vi "listMessageFiles.vi"(11 "folder Path":path) -> (1 "All Files in Dir":path[](array[path])=[path "/Volumes/CentralDataCache/2021/GDW-Metadata/metadata/Logs/Logs_01-2021/01-01/D01-Messages.xls", path "/Volumes/CentralDataCache/2021/GDW-Metadata/metadata/Logs/Logs_01-2021/02-01/D02-Messages.xls", path "/Volumes/CentralDataCache/2021/GDW-Metadata/metadata/Logs/Logs_01-2021/03-01/D03-Messages.xls", path "/Volumes/CentralDataCache/2021/GDW-Metadata/metadata/Logs/Logs_01-2021/04-01/D04-Messages.xls", path "/Volumes/CentralDataCache/2021/GDW-Metadata/metadata/Logs/Logs_01-2021/05-01/D05-Messages.xls", path "/Volumes/CentralDataCache/2021/GDW-Metadata/metadata/Logs/Logs_01-2021/06-01/D06-Messages.xls", path "/Volumes/CentralDataCache/2021/GDW-Metadata/metadata/Logs/Logs_01-2021/07-01/D07-Messages.xls", path "/Volumes/CentralDataCache/2021/GDW-Metadata/metadata/Logs/Logs_01-2021/08-01/D08-Messages.xls", path "/Volumes/CentralDataCache/2021/GDW-Metadata/metadata/Logs/Logs_01-2021/09-01/D09-Messages.xls", path "/Volumes/CentralDataCache/2021/GDW-Metadata/metadata/Logs/Logs_01-2021/10-01/D10-Messages.xls", path "/Volumes/CentralDataCache/2021/GDW-Metadata/metadata/Logs/Logs_01-2021/11-01/D11-Messages.xls", path "/Volumes/CentralDataCache/2021/GDW-Metadata/metadata/Logs/Logs_01-2021/12-01/D12-Messages.xls", path "/Volumes/CentralDataCache/2021/GDW-Metadata/metadata/Logs/Logs_01-2021/13-01/D13-Messages.xls", path "/Volumes/CentralDataCache/2021/GDW-Metadata/metadata/Logs/Logs_01-2021/14-01/D14-Messages.xls", path "/Volumes/CentralDataCache/2021/GDW-Metadata/metadata/Logs/Logs_01-2021/15-01/D15-Messages.xls", path "/Volumes/CentralDataCache/2021/GDW-Metadata/metadata/Logs/Logs_01-2021/16-01/D16-Messages.xls", path "/Volumes/CentralDataCache/2021/GDW-Metadata/metadata/Logs/Logs_01-2021/17-01/D17-Messages.xls", path "/Volumes/CentralDataCache/2021/GDW-Metadata/metadata/Logs/Logs_01-2021/18-01/D18-Messages.xls", path "/Volumes/CentralDataCache/2021/GDW-Metadata/metadata/Logs/Logs_01-2021/19-01/D19-Messages.xls", path "/Volumes/CentralDataCache/2021/GDW-Metadata/metadata/Logs/Logs_01-2021/20-01/D20-Messages.xls", path "/Volumes/CentralDataCache/2021/GDW-Metadata/metadata/Logs/Logs_01-2021/21-01/D21-Messages.xls", path "/Volumes/CentralDataCache/2021/GDW-Metadata/metadata/Logs/Logs_01-2021/22-01/D22-Messages.xls", path "/Volumes/CentralDataCache/2021/GDW-Metadata/metadata/Logs/Logs_01-2021/23-01/D23-Messages.xls", path "/Volumes/CentralDataCache/2021/GDW-Metadata/metadata/Logs/Logs_01-2021/24-01/D24-Messages.xls", path "/Volumes/CentralDataCache/2021/GDW-Metadata/metadata/Logs/Logs_01-2021/25-01/D25-Messages.xls", path "/Volumes/CentralDataCache/2021/GDW-Metadata/metadata/Logs/Logs_01-2021/26-01/D26-Messages.xls", path "/Volumes/CentralDataCache/2021/GDW-Metadata/metadata/Logs/Logs_01-2021/27-01/D27-Messages.xls", path "/Volumes/CentralDataCache/2021/GDW-Metadata/metadata/Logs/Logs_01-2021/28-01/D28-Messages.xls", path "/Volumes/CentralDataCache/2021/GDW-Metadata/metadata/Logs/Logs_01-2021/29-01/D29-Messages.xls", path "/Volumes/CentralDataCache/2021/GDW-Metadata/metadata/Logs/Logs_01-2021/30-01/D30-Messages.xls", path "/Volumes/CentralDataCache/2021/GDW-Metadata/metadata/Logs/Logs_01-2021/31-01/D31-Messages.xls", path "/Volumes/CentralDataCache/2021/GDW-Metadata/metadata/Logs/Logs_02-2021/01-02/D01-Messages.xls", path "/Volumes/CentralDataCache/2021/GDW-Metadata/metadata/Logs/Logs_02-2021/02-02/D02-Messages.xls", path "/Volumes/CentralDataCache/2021/GDW-Metadata/metadata/Logs/Logs_02-2021/03-02/D03-Messages.xls", path "/Volumes/CentralDataCache/2021/GDW-Metadata/metadata/Logs/Logs_02-2021/04-02/D04-Messages.xls", path "/Volumes/CentralDataCache/2021/GDW-Metadata/metadata/Logs/Logs_02-2021/05-02/D05-Messages.xls", path "/Volumes/CentralDataCache/2021/GDW-Metadata/metadata/Logs/Logs_02-2021/06-02/D06-Messages.xls", path "/Volumes/CentralDataCache/2021/GDW-Metadata/metadata/Logs/Logs_02-2021/07-02/D07-Messages.xls", path "/Volumes/CentralDataCache/2021/GDW-Metadata/metadata/Logs/Logs_02-2021/08-02/D08-Messages.xls", path "/Volumes/CentralDataCache/2021/GDW-Metadata/metadata/Logs/Logs_02-2021/09-02/D09-Messages.xls", path "/Volumes/CentralDataCache/2021/GDW-Metadata/metadata/Logs/Logs_02-2021/10-02/D10-Messages.xls", path "/Volumes/CentralDataCache/2021/GDW-Metadata/metadata/Logs/Logs_02-2021/11-02/D11-Messages.xls", path "/Volumes/CentralDataCache/2021/GDW-Metadata/metadata/Logs/Logs_02-2021/12-02/D12-Messages.xls", path "/Volumes/CentralDataCache/2021/GDW-Metadata/metadata/Logs/Logs_02-2021/13-02/D13-Messages.xls", path "/Volumes/CentralDataCache/2021/GDW-Metadata/metadata/Logs/Logs_02-2021/14-02/D14-Messages.xls", path "/Volumes/CentralDataCache/2021/GDW-Metadata/metadata/Logs/Logs_02-2021/15-02/D15-Messages.xls", path "/Volumes/CentralDataCache/2021/GDW-Metadata/metadata/Logs/Logs_02-2021/16-02/D16-Messages.xls", path "/Volumes/CentralDataCache/2021/GDW-Metadata/metadata/Logs/Logs_02-2021/17-02/D17-Messages.xls", path "/Volumes/CentralDataCache/2021/GDW-Metadata/metadata/Logs/Logs_02-2021/18-02/D18-Messages.xls", path "/Volumes/CentralDataCache/2021/GDW-Metadata/metadata/Logs/Logs_02-2021/19-02/D19-Messages.xls", path "/Volumes/CentralDataCache/2021/GDW-Metadata/metadata/Logs/Logs_02-2021/20-02/D20-Messages.xls", path "/Volumes/CentralDataCache/2021/GDW-Metadata/metadata/Logs/Logs_02-2021/21-02/D21-Messages.xls", path "/Volumes/CentralDataCache/2021/GDW-Metadata/metadata/Logs/Logs_02-2021/22-02/D22-Messages.xls", path "/Volumes/CentralDataCache/2021/GDW-Metadata/metadata/Logs/Logs_02-2021/23-02/D23-Messages.xls", path "/Volumes/CentralDataCache/2021/GDW-Metadata/metadata/Logs/Logs_02-2021/24-02/D24-Messages.xls", path "/Volumes/CentralDataCache/2021/GDW-Metadata/metadata/Logs/Logs_02-2021/25-02/D25-Messages.xls", path "/Volumes/CentralDataCache/2021/GDW-Metadata/metadata/Logs/Logs_02-2021/26-02/D26-Messages.xls", path "/Volumes/CentralDataCache/2021/GDW-Metadata/metadata/Logs/Logs_02-2021/27-02/D27-Messages.xls", path "/Volumes/CentralDataCache/2021/GDW-Metadata/metadata/Logs/Logs_02-2021/28-02/D28-Messages.xls", path "/Volumes/CentralDataCache/2021/GDW-Metadata/metadata/Logs/Logs_03-2021/01-03/D01-Messages.xls", path "/Volumes/CentralDataCache/2021/GDW-Metadata/metadata/Logs/Logs_03-2021/02-03/D02-Messages.xls", path "/Volumes/CentralDataCache/2021/GDW-Metadata/metadata/Logs/Logs_03-2021/03-03/D03-Messages.xls", path "/Volumes/CentralDataCache/2021/GDW-Metadata/metadata/Logs/Logs_03-2021/04-03/D04-Messages.xls", path "/Volumes/CentralDataCache/2021/GDW-Metadata/metadata/Logs/Logs_03-2021/05-03/D05-Messages.xls", path "/Volumes/CentralDataCache/2021/GDW-Metadata/metadata/Logs/Logs_03-2021/06-03/D06-Messages.xls", path "/Volumes/CentralDataCache/2021/GDW-Metadata/metadata/Logs/Logs_03-2021/07-03/D07-Messages.xls", path "/Volumes/CentralDataCache/2021/GDW-Metadata/metadata/Logs/Logs_03-2021/08-03/D08-Messages.xls", path "/Volumes/CentralDataCache/2021/GDW-Metadata/metadata/Logs/Logs_03-2021/09-03/D09-Messages.xls", path "/Volumes/CentralDataCache/2021/GDW-Metadata/metadata/Logs/Logs_03-2021/10-03/D10-Messages.xls", path "/Volumes/CentralDataCache/2021/GDW-Metadata/metadata/Logs/Logs_03-2021/11-03/D11-Messages.xls", path "/Volumes/CentralDataCache/2021/GDW-Metadata/metadata/Logs/Logs_03-2021/12-03/D12-Messages.xls", path "/Volumes/CentralDataCache/2021/GDW-Metadata/metadata/Logs/Logs_03-2021/13-03/D13-Messages.xls", path "/Volumes/CentralDataCache/2021/GDW-Metadata/metadata/Logs/Logs_03-2021/14-03/D14-Messages.xls", path "/Volumes/CentralDataCache/2021/GDW-Metadata/metadata/Logs/Logs_03-2021/15-03/D15-Messages.xls", path "/Volumes/CentralDataCache/2021/GDW-Metadata/metadata/Logs/Logs_03-2021/16-03/D16-Messages.xls", path "/Volumes/CentralDataCache/2021/GDW-Metadata/metadata/Logs/Logs_03-2021/17-03/D17-Messages.xls", path "/Volumes/CentralDataCache/2021/GDW-Metadata/metadata/Logs/Logs_03-2021/18-03/D18-Messages.xls", path "/Volumes/CentralDataCache/2021/GDW-Metadata/metadata/Logs/Logs_03-2021/19-03/D19-Messages.xls", path "/Volumes/CentralDataCache/2021/GDW-Metadata/metadata/Logs/Logs_03-2021/20-03/D20-Messages.xls", path "/Volumes/CentralDataCache/2021/GDW-Metadata/metadata/Logs/Logs_03-2021/21-03/D21-Messages.xls", path "/Volumes/CentralDataCache/2021/GDW-Metadata/metadata/Logs/Logs_03-2021/22-03/D22-Messages.xls", path "/Volumes/CentralDataCache/2021/GDW-Metadata/metadata/Logs/Logs_03-2021/23-03/D23-Messages.xls", path "/Volumes/CentralDataCache/2021/GDW-Metadata/metadata/Logs/Logs_03-2021/24-03/D24-Messages.xls", path "/Volumes/CentralDataCache/2021/GDW-Metadata/metadata/Logs/Logs_03-2021/25-03/D25-Messages.xls", path "/Volumes/CentralDataCache/2021/GDW-Metadata/metadata/Logs/Logs_03-2021/26-03/D26-Messages.xls", path "/Volumes/CentralDataCache/2021/GDW-Metadata/metadata/Logs/Logs_03-2021/27-03/D27-Messages.xls", path "/Volumes/CentralDataCache/2021/GDW-Metadata/metadata/Logs/Logs_03-2021/29-03/D29-Messages.xls", path "/Volumes/CentralDataCache/2021/GDW-Metadata/metadata/Logs/Logs_03-2021/30-03/D30-Messages.xls", path "/Volumes/CentralDataCache/2021/GDW-Metadata/metadata/Logs/Logs_03-2021/31-03/D31-Messages.xls", path "/Volumes/CentralDataCache/2021/GDW-Metadata/metadata/Logs/Logs_04-2021/01-04/D01-Messages.xls", path "/Volumes/CentralDataCache/2021/GDW-Metadata/metadata/Logs/Logs_04-2021/02-04/D02-Messages.xls", path "/Volumes/CentralDataCache/2021/GDW-Metadata/metadata/Logs/Logs_04-2021/03-04/D03-Messages.xls", path "/Volumes/CentralDataCache/2021/GDW-Metadata/metadata/Logs/Logs_04-2021/04-04/D04-Messages.xls", path "/Volumes/CentralDataCache/2021/GDW-Metadata/metadata/Logs/Logs_04-2021/05-04/D05-Messages.xls", path "/Volumes/CentralDataCache/2021/GDW-Metadata/metadata/Logs/Logs_04-2021/06-04/D06-Messages.xls", path "/Volumes/CentralDataCache/2021/GDW-Metadata/metadata/Logs/Logs_04-2021/07-04/D07-Messages.xls", path "/Volumes/CentralDataCache/2021/GDW-Metadata/metadata/Logs/Logs_04-2021/08-04/D08-Messages.xls", path "/Volumes/CentralDataCache/2021/GDW-Metadata/metadata/Logs/Logs_04-2021/09-04/D09-Messages.xls", path "/Volumes/CentralDataCache/2021/GDW-Metadata/metadata/Logs/Logs_04-2021/10-04/D10-Messages.xls", path "/Volumes/CentralDataCache/2021/GDW-Metadata/metadata/Logs/Logs_04-2021/11-04/D11-Messages.xls", path "/Volumes/CentralDataCache/2021/GDW-Metadata/metadata/Logs/Logs_04-2021/12-04/D12-Messages.xls", path "/Volumes/CentralDataCache/2021/GDW-Metadata/metadata/Logs/Logs_04-2021/13-04/D13-Messages.xls", path "/Volumes/CentralDataCache/2021/GDW-Metadata/metadata/Logs/Logs_04-2021/14-04/D14-Messages.xls", path "/Volumes/CentralDataCache/2021/GDW-Metadata/metadata/Logs/Logs_04-2021/15-04/D15-Messages.xls", path "/Volumes/CentralDataCache/2021/GDW-Metadata/metadata/Logs/Logs_04-2021/16-04/D16-Messages.xls", path "/Volumes/CentralDataCache/2021/GDW-Metadata/metadata/Logs/Logs_04-2021/17-04/D17-Messages.xls", path "/Volumes/CentralDataCache/2021/GDW-Metadata/metadata/Logs/Logs_04-2021/18-04/D18-Messages.xls", path "/Volumes/CentralDataCache/2021/GDW-Metadata/metadata/Logs/Logs_04-2021/19-04/D19-Messages.xls", path "/Volumes/CentralDataCache/2021/GDW-Metadata/metadata/Logs/Logs_04-2021/20-04/D20-Messages.xls", path "/Volumes/CentralDataCache/2021/GDW-Metadata/metadata/Logs/Logs_04-2021/21-04/D21-Messages.xls", path "/Volumes/CentralDataCache/2021/GDW-Metadata/metadata/Logs/Logs_04-2021/22-04/D22-Messages.xls", path "/Volumes/CentralDataCache/2021/GDW-Metadata/metadata/Logs/Logs_04-2021/23-04/D23-Messages.xls", path "/Volumes/CentralDataCache/2021/GDW-Metadata/metadata/Logs/Logs_04-2021/24-04/D24-Messages.xls", path "/Volumes/CentralDataCache/2021/GDW-Metadata/metadata/Logs/Logs_04-2021/25-04/D25-Messages.xls", path "/Volumes/CentralDataCache/2021/GDW-Metadata/metadata/Logs/Logs_04-2021/26-04/D26-Messages.xls", path "/Volumes/CentralDataCache/2021/GDW-Metadata/metadata/Logs/Logs_04-2021/27-04/D27-Messages.xls", path "/Volumes/CentralDataCache/2021/GDW-Metadata/metadata/Logs/Logs_04-2021/28-04/D28-Messages.xls", path "/Volumes/CentralDataCache/2021/GDW-Metadata/metadata/Logs/Logs_04-2021/29-04/D29-Messages.xls", path "/Volumes/CentralDataCache/2021/GDW-Metadata/metadata/Logs/Logs_04-2021/30-04/D30-Messages.xls", path "/Volumes/CentralDataCache/2021/GDW-Metadata/metadata/Logs/Logs_05-2021/01-05/D01-Messages.xls", path "/Volumes/CentralDataCache/2021/GDW-Metadata/metadata/Logs/Logs_05-2021/02-05/D02-Messages.xls", path "/Volumes/CentralDataCache/2021/GDW-Metadata/metadata/Logs/Logs_05-2021/03-05/D03-Messages.xls", path "/Volumes/CentralDataCache/2021/GDW-Metadata/metadata/Logs/Logs_05-2021/04-05/D04-Messages.xls", path "/Volumes/CentralDataCache/2021/GDW-Metadata/metadata/Logs/Logs_05-2021/05-05/D05-Messages.xls", path "/Volumes/CentralDataCache/2021/GDW-Metadata/metadata/Logs/Logs_05-2021/06-05/D06-Messages.xls", path "/Volumes/CentralDataCache/2021/GDW-Metadata/metadata/Logs/Logs_05-2021/07-05/D07-Messages.xls", path "/Volumes/CentralDataCache/2021/GDW-Metadata/metadata/Logs/Logs_05-2021/08-05/D08-Messages.xls", path "/Volumes/CentralDataCache/2021/GDW-Metadata/metadata/Logs/Logs_05-2021/09-05/D09-Messages.xls", path "/Volumes/CentralDataCache/2021/GDW-Metadata/metadata/Logs/Logs_05-2021/10-05/D10-Messages.xls", path "/Volumes/CentralDataCache/2021/GDW-Metadata/metadata/Logs/Logs_05-2021/11-05/D11-Messages.xls", path "/Volumes/CentralDataCache/2021/GDW-Metadata/metadata/Logs/Logs_05-2021/12-05/D12-Messages.xls", path "/Volumes/CentralDataCache/2021/GDW-Metadata/metadata/Logs/Logs_05-2021/13-05/D13-Messages.xls", path "/Volumes/CentralDataCache/2021/GDW-Metadata/metadata/Logs/Logs_05-2021/14-05/D14-Messages.xls", path "/Volumes/CentralDataCache/2021/GDW-Metadata/metadata/Logs/Logs_05-2021/15-05/D15-Messages.xls", path "/Volumes/CentralDataCache/2021/GDW-Metadata/metadata/Logs/Logs_05-2021/16-05/D16-Messages.xls", path "/Volumes/CentralDataCache/2021/GDW-Metadata/metadata/Logs/Logs_05-2021/17-05/D17-Messages.xls", path "/Volumes/CentralDataCache/2021/GDW-Metadata/metadata/Logs/Logs_05-2021/18-05/D18-Messages.xls", path "/Volumes/CentralDataCache/2021/GDW-Metadata/metadata/Logs/Logs_05-2021/19-05/D19-Messages.xls", path "/Volumes/CentralDataCache/2021/GDW-Metadata/metadata/Logs/Logs_05-2021/20-05/D20-Messages.xls", path "/Volumes/CentralDataCache/2021/GDW-Metadata/metadata/Logs/Logs_05-2021/21-05/D21-Messages.xls", path "/Volumes/CentralDataCache/2021/GDW-Metadata/metadata/Logs/Logs_05-2021/22-05/D22-Messages.xls", path "/Volumes/CentralDataCache/2021/GDW-Metadata/metadata/Logs/Logs_05-2021/23-05/D23-Messages.xls", path "/Volumes/CentralDataCache/2021/GDW-Metadata/metadata/Logs/Logs_05-2021/24-05/D24-Messages.xls", path "/Volumes/CentralDataCache/2021/GDW-Metadata/metadata/Logs/Logs_05-2021/25-05/D25-Messages.xls", path "/Volumes/CentralDataCache/2021/GDW-Metadata/metadata/Logs/Logs_05-2021/26-05/D26-Messages.xls", path "/Volumes/CentralDataCache/2021/GDW-Metadata/metadata/Logs/Logs_05-2021/27-05/D27-Messages.xls", path "/Volumes/CentralDataCache/2021/GDW-Metadata/metadata/Logs/Logs_05-2021/28-05/D28-Messages.xls", path "/Volumes/CentralDataCache/2021/GDW-Metadata/metadata/Logs/Logs_05-2021/29-05/D29-Messages.xls", path "/Volumes/CentralDataCache/2021/GDW-Metadata/metadata/Logs/Logs_05-2021/30-05/D30-Messages.xls", path "/Volumes/CentralDataCache/2021/GDW-Metadata/metadata/Logs/Logs_05-2021/31-05/D31-Messages.xls", path "/Volumes/CentralDataCache/2021/GDW-Metadata/metadata/Logs/Logs_06-2021/01-06/D01-Messages.xls", path "/Volumes/CentralDataCache/2021/GDW-Metadata/metadata/Logs/Logs_06-2021/02-06/D02-Messages.xls", path "/Volumes/CentralDataCache/2021/GDW-Metadata/metadata/Logs/Logs_06-2021/03-06/D03-Messages.xls", path "/Volumes/CentralDataCache/2021/GDW-Metadata/metadata/Logs/Logs_06-2021/04-06/D04-Messages.xls", path "/Volumes/CentralDataCache/2021/GDW-Metadata/metadata/Logs/Logs_06-2021/05-06/D05-Messages.xls", path "/Volumes/CentralDataCache/2021/GDW-Metadata/metadata/Logs/Logs_06-2021/06-06/D06-Messages.xls", path "/Volumes/CentralDataCache/2021/GDW-Metadata/metadata/Logs/Logs_06-2021/07-06/D07-Messages.xls", path "/Volumes/CentralDataCache/2021/GDW-Metadata/metadata/Logs/Logs_06-2021/08-06/D08-Messages.xls", path "/Volumes/CentralDataCache/2021/GDW-Metadata/metadata/Logs/Logs_06-2021/09-06/D09-Messages.xls", path "/Volumes/CentralDataCache/2021/GDW-Metadata/metadata/Logs/Logs_06-2021/10-06/D10-Messages.xls", path "/Volumes/CentralDataCache/2021/GDW-Metadata/metadata/Logs/Logs_06-2021/11-06/D11-Messages.xls", path "/Volumes/CentralDataCache/2021/GDW-Metadata/metadata/Logs/Logs_06-2021/12-06/D12-Messages.xls", path "/Volumes/CentralDataCache/2021/GDW-Metadata/metadata/Logs/Logs_06-2021/13-06/D13-Messages.xls", path "/Volumes/CentralDataCache/2021/GDW-Metadata/metadata/Logs/Logs_06-2021/14-06/D14-Messages.xls", path "/Volumes/CentralDataCache/2021/GDW-Metadata/metadata/Logs/Logs_06-2021/15-06/D15-Messages.xls", path "/Volumes/CentralDataCache/2021/GDW-Metadata/metadata/Logs/Logs_06-2021/16-06/D16-Messages.xls", path "/Volumes/CentralDataCache/2021/GDW-Metadata/metadata/Logs/Logs_06-2021/17-06/D17-Messages.xls", path "/Volumes/CentralDataCache/2021/GDW-Metadata/metadata/Logs/Logs_06-2021/18-06/D18-Messages.xls", path "/Volumes/CentralDataCache/2021/GDW-Metadata/metadata/Logs/Logs_06-2021/19-06/D19-Messages.xls", path "/Volumes/CentralDataCache/2021/GDW-Metadata/metadata/Logs/Logs_06-2021/20-06/D20-Messages.xls", path "/Volumes/CentralDataCache/2021/GDW-Metadata/metadata/Logs/Logs_06-2021/21-06/D21-Messages.xls", path "/Volumes/CentralDataCache/2021/GDW-Metadata/metadata/Logs/Logs_06-2021/22-06/D22-Messages.xls", path "/Volumes/CentralDataCache/2021/GDW-Metadata/metadata/Logs/Logs_06-2021/23-06/D23-Messages.xls", path "/Volumes/CentralDataCache/2021/GDW-Metadata/metadata/Logs/Logs_06-2021/24-06/D24-Messages.xls", path "/Volumes/CentralDataCache/2021/GDW-Metadata/metadata/Logs/Logs_06-2021/25-06/D25-Messages.xls", path "/Volumes/CentralDataCache/2021/GDW-Metadata/metadata/Logs/Logs_06-2021/26-06/D26-Messages.xls", path "/Volumes/CentralDataCache/2021/GDW-Metadata/metadata/Logs/Logs_06-2021/27-06/D27-Messages.xls", path "/Volumes/CentralDataCache/2021/GDW-Metadata/metadata/Logs/Logs_06-2021/28-06/D28-Messages.xls", path "/Volumes/CentralDataCache/2021/GDW-Metadata/metadata/Logs/Logs_06-2021/29-06/D29-Messages.xls", path "/Volumes/CentralDataCache/2021/GDW-Metadata/metadata/Logs/Logs_06-2021/30-06/D30-Messages.xls", path "/Volumes/CentralDataCache/2021/GDW-Metadata/metadata/Logs/Logs_07-2021/01-07/D01-Messages.xls", path "/Volumes/CentralDataCache/2021/GDW-Metadata/metadata/Logs/Logs_07-2021/02-07/D02-Messages.xls", path "/Volumes/CentralDataCache/2021/GDW-Metadata/metadata/Logs/Logs_07-2021/03-07/D03-Messages.xls", path "/Volumes/CentralDataCache/2021/GDW-Metadata/metadata/Logs/Logs_07-2021/04-07/D04-Messages.xls", path "/Volumes/CentralDataCache/2021/GDW-Metadata/metadata/Logs/Logs_07-2021/05-07/D05-Messages.xls", path "/Volumes/CentralDataCache/2021/GDW-Metadata/metadata/Logs/Logs_07-2021/06-07/D06-Messages.xls", path "/Volumes/CentralDataCache/2021/GDW-Metadata/metadata/Logs/Logs_07-2021/07-07/D07-Messages.xls", path "/Volumes/CentralDataCache/2021/GDW-Metadata/metadata/Logs/Logs_07-2021/08-07/D08-Messages.xls", path "/Volumes/CentralDataCache/2021/GDW-Metadata/metadata/Logs/Logs_07-2021/09-07/D09-Messages.xls", path "/Volumes/CentralDataCache/2021/GDW-Metadata/metadata/Logs/Logs_07-2021/10-07/D10-Messages.xls", path "/Volumes/CentralDataCache/2021/GDW-Metadata/metadata/Logs/Logs_07-2021/11-07/D11-Messages.xls", path "/Volumes/CentralDataCache/2021/GDW-Metadata/metadata/Logs/Logs_07-2021/12-07/D12-Messages.xls", path "/Volumes/CentralDataCache/2021/GDW-Metadata/metadata/Logs/Logs_07-2021/13-07/D13-Messages.xls", path "/Volumes/CentralDataCache/2021/GDW-Metadata/metadata/Logs/Logs_07-2021/14-07/D14-Messages.xls", path "/Volumes/CentralDataCache/2021/GDW-Metadata/metadata/Logs/Logs_07-2021/15-07/D15-Messages.xls", path "/Volumes/CentralDataCache/2021/GDW-Metadata/metadata/Logs/Logs_07-2021/16-07/D16-Messages.xls", path "/Volumes/CentralDataCache/2021/GDW-Metadata/metadata/Logs/Logs_07-2021/17-07/D17-Messages.xls", path "/Volumes/CentralDataCache/2021/GDW-Metadata/metadata/Logs/Logs_07-2021/18-07/D18-Messages.xls", path "/Volumes/CentralDataCache/2021/GDW-Metadata/metadata/Logs/Logs_07-2021/19-07/D19-Messages.xls", path "/Volumes/CentralDataCache/2021/GDW-Metadata/metadata/Logs/Logs_07-2021/20-07/D20-Messages.xls", path "/Volumes/CentralDataCache/2021/GDW-Metadata/metadata/Logs/Logs_07-2021/21-07/D21-Messages.xls", path "/Volumes/CentralDataCache/2021/GDW-Metadata/metadata/Logs/Logs_07-2021/22-07/D22-Messages.xls", path "/Volumes/CentralDataCache/2021/GDW-Metadata/metadata/Logs/Logs_07-2021/23-07/D23-Messages.xls", path "/Volumes/CentralDataCache/2021/GDW-Metadata/metadata/Logs/Logs_07-2021/24-07/D24-Messages.xls", path "/Volumes/CentralDataCache/2021/GDW-Metadata/metadata/Logs/Logs_07-2021/25-07/D25-Messages.xls", path "/Volumes/CentralDataCache/2021/GDW-Metadata/metadata/Logs/Logs_07-2021/26-07/D26-Messages.xls", path "/Volumes/CentralDataCache/2021/GDW-Metadata/metadata/Logs/Logs_07-2021/27-07/D27-Messages.xls", path "/Volumes/CentralDataCache/2021/GDW-Metadata/metadata/Logs/Logs_07-2021/28-07/D28-Messages.xls", path "/Volumes/CentralDataCache/2021/GDW-Metadata/metadata/Logs/Logs_07-2021/29-07/D29-Messages.xls", path "/Volumes/CentralDataCache/2021/GDW-Metadata/metadata/Logs/Logs_07-2021/30-07/D30-Messages.xls", path "/Volumes/CentralDataCache/2021/GDW-Metadata/metadata/Logs/Logs_07-2021/31-07/D31-Messages.xls", path "/Volumes/CentralDataCache/2021/GDW-Metadata/metadata/Logs/Logs_08-2021/01-08/D01-Messages.xls", path "/Volumes/CentralDataCache/2021/GDW-Metadata/metadata/Logs/Logs_08-2021/02-08/D02-Messages.xls", path "/Volumes/CentralDataCache/2021/GDW-Metadata/metadata/Logs/Logs_08-2021/03-08/D03-Messages.xls", path "/Volumes/CentralDataCache/2021/GDW-Metadata/metadata/Logs/Logs_08-2021/04-08/D04-Messages.xls", path "/Volumes/CentralDataCache/2021/GDW-Metadata/metadata/Logs/Logs_08-2021/05-08/D05-Messages.xls", path "/Volumes/CentralDataCache/2021/GDW-Metadata/metadata/Logs/Logs_08-2021/06-08/D06-Messages.xls", path "/Volumes/CentralDataCache/2021/GDW-Metadata/metadata/Logs/Logs_08-2021/07-08/D07-Messages.xls", path "/Volumes/CentralDataCache/2021/GDW-Metadata/metadata/Logs/Logs_08-2021/08-08/D08-Messages.xls", path "/Volumes/CentralDataCache/2021/GDW-Metadata/metadata/Logs/Logs_08-2021/09-08/D09-Messages.xls", path "/Volumes/CentralDataCache/2021/GDW-Metadata/metadata/Logs/Logs_08-2021/10-08/D10-Messages.xls", path "/Volumes/CentralDataCache/2021/GDW-Metadata/metadata/Logs/Logs_08-2021/11-08/D11-Messages.xls", path "/Volumes/CentralDataCache/2021/GDW-Metadata/metadata/Logs/Logs_08-2021/12-08/D12-Messages.xls", path "/Volumes/CentralDataCache/2021/GDW-Metadata/metadata/Logs/Logs_08-2021/13-08/D13-Messages.xls", path "/Volumes/CentralDataCache/2021/GDW-Metadata/metadata/Logs/Logs_08-2021/17-08/D17-Messages.xls", path "/Volumes/CentralDataCache/2021/GDW-Metadata/metadata/Logs/Logs_08-2021/18-08/D18-Messages.xls", path "/Volumes/CentralDataCache/2021/GDW-Metadata/metadata/Logs/Logs_08-2021/19-08/D19-Messages.xls", path "/Volumes/CentralDataCache/2021/GDW-Metadata/metadata/Logs/Logs_08-2021/20-08/D20-Messages.xls", path "/Volumes/CentralDataCache/2021/GDW-Metadata/metadata/Logs/Logs_08-2021/21-08/D21-Messages.xls", path "/Volumes/CentralDataCache/2021/GDW-Metadata/metadata/Logs/Logs_08-2021/22-08/D22-Messages.xls", path "/Volumes/CentralDataCache/2021/GDW-Metadata/metadata/Logs/Logs_08-2021/23-08/D23-Messages.xls", path "/Volumes/CentralDataCache/2021/GDW-Metadata/metadata/Logs/Logs_08-2021/24-08/D24-Messages.xls", path "/Volumes/CentralDataCache/2021/GDW-Metadata/metadata/Logs/Logs_08-2021/25-08/D25-Messages.xls", path "/Volumes/CentralDataCache/2021/GDW-Metadata/metadata/Logs/Logs_08-2021/26-08/D26-Messages.xls", path "/Volumes/CentralDataCache/2021/GDW-Metadata/metadata/Logs/Logs_08-2021/27-08/D27-Messages.xls", path "/Volumes/CentralDataCache/2021/GDW-Metadata/metadata/Logs/Logs_08-2021/28-08/D28-Messages.xls", path "/Volumes/CentralDataCache/2021/GDW-Metadata/metadata/Logs/Logs_08-2021/29-08/D29-Messages.xls", path "/Volumes/CentralDataCache/2021/GDW-Metadata/metadata/Logs/Logs_08-2021/30-08/D30-Messages.xls", path "/Volumes/CentralDataCache/2021/GDW-Metadata/metadata/Logs/Logs_08-2021/31-08/D31-Messages.xls", path "/Volumes/CentralDataCache/2021/GDW-Metadata/metadata/Logs/Logs_09-2021/01-09/D01-Messages.xls", path "/Volumes/CentralDataCache/2021/GDW-Metadata/metadata/Logs/Logs_09-2021/02-09/D02-Messages.xls", path "/Volumes/CentralDataCache/2021/GDW-Metadata/metadata/Logs/Logs_09-2021/03-09/D03-Messages.xls", path "/Volumes/CentralDataCache/2021/GDW-Metadata/metadata/Logs/Logs_09-2021/04-09/D04-Messages.xls", path "/Volumes/CentralDataCache/2021/GDW-Metadata/metadata/Logs/Logs_09-2021/05-09/D05-Messages.xls", path "/Volumes/CentralDataCache/2021/GDW-Metadata/metadata/Logs/Logs_09-2021/06-09/D06-Messages.xls", path "/Volumes/CentralDataCache/2021/GDW-Metadata/metadata/Logs/Logs_09-2021/07-09/D07-Messages.xls", path "/Volumes/CentralDataCache/2021/GDW-Metadata/metadata/Logs/Logs_09-2021/08-09/D08-Messages.xls", path "/Volumes/CentralDataCache/2021/GDW-Metadata/metadata/Logs/Logs_09-2021/09-09/D09-Messages.xls", path "/Volumes/CentralDataCache/2021/GDW-Metadata/metadata/Logs/Logs_09-2021/10-09/D10-Messages.xls", path "/Volumes/CentralDataCache/2021/GDW-Metadata/metadata/Logs/Logs_09-2021/11-09/D11-Messages.xls", path "/Volumes/CentralDataCache/2021/GDW-Metadata/metadata/Logs/Logs_09-2021/12-09/D12-Messages.xls", path "/Volumes/CentralDataCache/2021/GDW-Metadata/metadata/Logs/Logs_09-2021/13-09/D13-Messages.xls", path "/Volumes/CentralDataCache/2021/GDW-Metadata/metadata/Logs/Logs_09-2021/14-09/D14-Messages.xls", path "/Volumes/CentralDataCache/2021/GDW-Metadata/metadata/Logs/Logs_09-2021/15-09/D15-Messages.xls", path "/Volumes/CentralDataCache/2021/GDW-Metadata/metadata/Logs/Logs_09-2021/16-09/D16-Messages.xls", path "/Volumes/CentralDataCache/2021/GDW-Metadata/metadata/Logs/Logs_09-2021/17-09/D17-Messages.xls", path "/Volumes/CentralDataCache/2021/GDW-Metadata/metadata/Logs/Logs_09-2021/18-09/D18-Messages.xls", path "/Volumes/CentralDataCache/2021/GDW-Metadata/metadata/Logs/Logs_09-2021/19-09/D19-Messages.xls", path "/Volumes/CentralDataCache/2021/GDW-Metadata/metadata/Logs/Logs_09-2021/20-09/D20-Messages.xls", path "/Volumes/CentralDataCache/2021/GDW-Metadata/metadata/Logs/Logs_09-2021/21-09/D21-Messages.xls", path "/Volumes/CentralDataCache/2021/GDW-Metadata/metadata/Logs/Logs_09-2021/22-09/D22-Messages.xls", path "/Volumes/CentralDataCache/2021/GDW-Metadata/metadata/Logs/Logs_09-2021/23-09/D23-Messages.xls", path "/Volumes/CentralDataCache/2021/GDW-Metadata/metadata/Logs/Logs_09-2021/24-09/D24-Messages.xls", path "/Volumes/CentralDataCache/2021/GDW-Metadata/metadata/Logs/Logs_09-2021/25-09/D25-Messages.xls", path "/Volumes/CentralDataCache/2021/GDW-Metadata/metadata/Logs/Logs_09-2021/26-09/D26-Messages.xls", path "/Volumes/CentralDataCache/2021/GDW-Metadata/metadata/Logs/Logs_09-2021/27-09/D27-Messages.xls", path "/Volumes/CentralDataCache/2021/GDW-Metadata/metadata/Logs/Logs_09-2021/28-09/D28-Messages.xls", path "/Volumes/CentralDataCache/2021/GDW-Metadata/metadata/Logs/Logs_09-2021/29-09/D29-Messages.xls", path "/Volumes/CentralDataCache/2021/GDW-Metadata/metadata/Logs/Logs_09-2021/30-09/D30-Messages.xls", path "/Volumes/CentralDataCache/2021/GDW-Metadata/metadata/Logs/Logs_10-2021/01-10/D01-Messages.xls", path "/Volumes/CentralDataCache/2021/GDW-Metadata/metadata/Logs/Logs_10-2021/02-10/D02-Messages.xls", path "/Volumes/CentralDataCache/2021/GDW-Metadata/metadata/Logs/Logs_10-2021/03-10/D03-Messages.xls", path "/Volumes/CentralDataCache/2021/GDW-Metadata/metadata/Logs/Logs_10-2021/04-10/D04-Messages.xls", path "/Volumes/CentralDataCache/2021/GDW-Metadata/metadata/Logs/Logs_10-2021/05-10/D05-Messages.xls", path "/Volumes/CentralDataCache/2021/GDW-Metadata/metadata/Logs/Logs_10-2021/06-10/D06-Messages.xls", path "/Volumes/CentralDataCache/2021/GDW-Metadata/metadata/Logs/Logs_10-2021/07-10/D07-Messages.xls", path "/Volumes/CentralDataCache/2021/GDW-Metadata/metadata/Logs/Logs_10-2021/08-10/D08-Messages.xls", path "/Volumes/CentralDataCache/2021/GDW-Metadata/metadata/Logs/Logs_10-2021/09-10/D09-Messages.xls", path "/Volumes/CentralDataCache/2021/GDW-Metadata/metadata/Logs/Logs_10-2021/10-10/D10-Messages.xls", path "/Volumes/CentralDataCache/2021/GDW-Metadata/metadata/Logs/Logs_10-2021/11-10/D11-Messages.xls", path "/Volumes/CentralDataCache/2021/GDW-Metadata/metadata/Logs/Logs_10-2021/12-10/D12-Messages.xls", path "/Volumes/CentralDataCache/2021/GDW-Metadata/metadata/Logs/Logs_10-2021/13-10/D13-Messages.xls", path "/Volumes/CentralDataCache/2021/GDW-Metadata/metadata/Logs/Logs_10-2021/14-10/D14-Messages.xls", path "/Volumes/CentralDataCache/2021/GDW-Metadata/metadata/Logs/Logs_10-2021/15-10/D15-Messages.xls", path "/Volumes/CentralDataCache/2021/GDW-Metadata/metadata/Logs/Logs_10-2021/16-10/D16-Messages.xls", path "/Volumes/CentralDataCache/2021/GDW-Metadata/metadata/Logs/Logs_10-2021/17-10/D17-Messages.xls", path "/Volumes/CentralDataCache/2021/GDW-Metadata/metadata/Logs/Logs_10-2021/18-10/D18-Messages.xls", path "/Volumes/CentralDataCache/2021/GDW-Metadata/metadata/Logs/Logs_10-2021/19-10/D19-Messages.xls", path "/Volumes/CentralDataCache/2021/GDW-Metadata/metadata/Logs/Logs_10-2021/20-10/D20-Messages.xls", path "/Volumes/CentralDataCache/2021/GDW-Metadata/metadata/Logs/Logs_10-2021/21-10/D21-Messages.xls", path "/Volumes/CentralDataCache/2021/GDW-Metadata/metadata/Logs/Logs_10-2021/22-10/D22-Messages.xls", path "/Volumes/CentralDataCache/2021/GDW-Metadata/metadata/Logs/Logs_10-2021/23-10/D23-Messages.xls", path "/Volumes/CentralDataCache/2021/GDW-Metadata/metadata/Logs/Logs_10-2021/24-10/D24-Messages.xls", path "/Volumes/CentralDataCache/2021/GDW-Metadata/metadata/Logs/Logs_10-2021/25-10/D25-Messages.xls", path "/Volumes/CentralDataCache/2021/GDW-Metadata/metadata/Logs/Logs_10-2021/26-10/D26-Messages.xls"])   [LabVIEW 2020]
panel:
  in  "useCached":bool
  out "Number of Files":i32
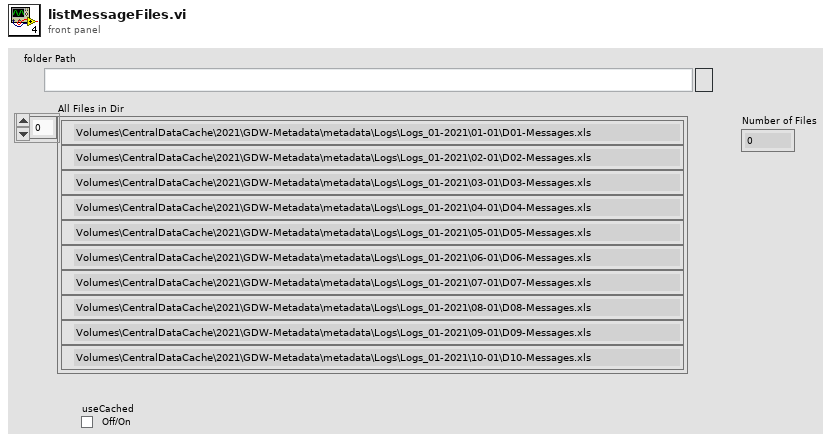
[diagram p1: front panel]
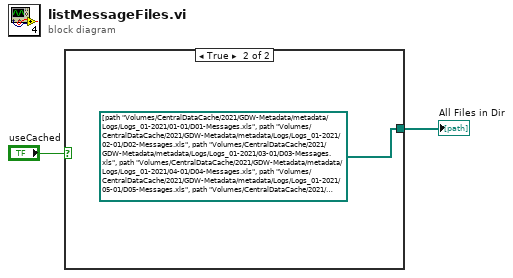
[diagram p0: block diagram]
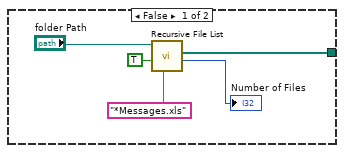
[diagram p2: hidden frame]
diagram:
  n1 = case shown="True" "useCached" {
    tunnel: [w4 path[] [path "/Volumes/CentralDataCache/2021/GDW-Metadata/metadata/Logs/Logs_01-2021/01-01/D01-Messages.xls", path "/Volumes/CentralDataCache/2021/GDW-Metadata/metadata/Logs/Logs_01-2021/02-01/D02-Messages.xls", path "/Volumes/CentralDataCache/2021/GDW-Metadata/metadata/Logs/Logs_01-2021/03-01/D03-Messages.xls", path "/Volumes/CentralDataCache/2021/GDW-Metadata/metadata/Logs/Logs_01-2021/04-01/D04-Messages.xls", path "/Volumes/CentralDataCache/2021/GDW-Metadata/metadata/Logs/Logs_01-2021/05-01/D05-Messages.xls", path "/Volumes/CentralDataCache/2021/GDW-Metadata/metadata/Logs/Logs_01-2021/06-01/D06-Messages.xls", path "/Volumes/CentralDataCache/2021/GDW-Metadata/metadata/Logs/Logs_01-2021/07-01/D07-Messages.xls", path "/Volumes/CentralDataCache/2021/GDW-Metadata/metadata/Logs/Logs_01-2021/08-01/D08-Messages.xls", path "/Volumes/CentralDataCache/2021/GDW-Metadata/metadata/Logs/Logs_01-2021/09-01/D09-Messages.xls", path "/Volumes/CentralDataCache/2021/GDW-Metadata/metadata/Logs/Logs_01-2021/10-01/D10-Messages.xls", path "/Volumes/CentralDataCache/2021/GDW-Metadata/metadata/Logs/Logs_01-2021/11-01/D11-Messages.xls", path "/Volumes/CentralDataCache/2021/GDW-Metadata/metadata/Logs/Logs_01-2021/12-01/D12-Messages.xls", path "/Volumes/CentralDataCache/2021/GDW-Metadata/metadata/Logs/Logs_01-2021/13-01/D13-Messages.xls", path "/Volumes/CentralDataCache/2021/GDW-Metadata/metadata/Logs/Logs_01-2021/14-01/D14-Messages.xls", path "/Volumes/CentralDataCache/2021/GDW-Metadata/metadata/Logs/Logs_01-2021/15-01/D15-Messages.xls", path "/Volumes/CentralDataCache/2021/GDW-Metadata/metadata/Logs/Logs_01-2021/16-01/D16-Messages.xls", path "/Volumes/CentralDataCache/2021/GDW-Metadata/metadata/Logs/Logs_01-2021/17-01/D17-Messages.xls", path "/Volumes/CentralDataCache/2021/GDW-Metadata/metadata/Logs/Logs_01-2021/18-01/D18-Messages.xls", path "/Volumes/CentralDataCache/2021/GDW-Metadata/metadata/Logs/Logs_01-2021/19-01/D19-Messages.xls", path "/Volumes/CentralDataCache/2021/GDW-Metadata/metadata/Logs/Logs_01-2021/20-01/D20-Messages.xls", path "/Volumes/CentralDataCache/2021/GDW-Metadata/metadata/Logs/Logs_01-2021/21-01/D21-Messages.xls", path "/Volumes/CentralDataCache/2021/GDW-Metadata/metadata/Logs/Logs_01-2021/22-01/D22-Messages.xls", path "/Volumes/CentralDataCache/2021/GDW-Metadata/metadata/Logs/Logs_01-2021/23-01/D23-Messages.xls", path "/Volumes/CentralDataCache/2021/GDW-Metadata/metadata/Logs/Logs_01-2021/24-01/D24-Messages.xls", path "/Volumes/CentralDataCache/2021/GDW-Metadata/metadata/Logs/Logs_01-2021/25-01/D25-Messages.xls", path "/Volumes/CentralDataCache/2021/GDW-Metadata/metadata/Logs/Logs_01-2021/26-01/D26-Messages.xls", path "/Volumes/CentralDataCache/2021/GDW-Metadata/metadata/Logs/Logs_01-2021/27-01/D27-Messages.xls", path "/Volumes/CentralDataCache/2021/GDW-Metadata/metadata/Logs/Logs_01-2021/28-01/D28-Messages.xls", path "/Volumes/CentralDataCache/2021/GDW-Metadata/metadata/Logs/Logs_01-2021/29-01/D29-Messages.xls", path "/Volumes/CentralDataCache/2021/GDW-Metadata/metadata/Logs/Logs_01-2021/30-01/D30-Messages.xls", path "/Volumes/CentralDataCache/2021/GDW-Metadata/metadata/Logs/Logs_01-2021/31-01/D31-Messages.xls", path "/Volumes/CentralDataCache/2021/GDW-Metadata/metadata/Logs/Logs_02-2021/01-02/D01-Messages.xls", path "/Volumes/CentralDataCache/2021/GDW-Metadata/metadata/Logs/Logs_02-2021/02-02/D02-Messages.xls", path "/Volumes/CentralDataCache/2021/GDW-Metadata/metadata/Logs/Logs_02-2021/03-02/D03-Messages.xls", path "/Volumes/CentralDataCache/2021/GDW-Metadata/metadata/Logs/Logs_02-2021/04-02/D04-Messages.xls", path "/Volumes/CentralDataCache/2021/GDW-Metadata/metadata/Logs/Logs_02-2021/05-02/D05-Messages.xls", path "/Volumes/CentralDataCache/2021/GDW-Metadata/metadata/Logs/Logs_02-2021/06-02/D06-Messages.xls", path "/Volumes/CentralDataCache/2021/GDW-Metadata/metadata/Logs/Logs_02-2021/07-02/D07-Messages.xls", path "/Volumes/CentralDataCache/2021/GDW-Metadata/metadata/Logs/Logs_02-2021/08-02/D08-Messages.xls", path "/Volumes/CentralDataCache/2021/GDW-Metadata/metadata/Logs/Logs_02-2021/09-02/D09-Messages.xls", path "/Volumes/CentralDataCache/2021/GDW-Metadata/metadata/Logs/Logs_02-2021/10-02/D10-Messages.xls", path "/Volumes/CentralDataCache/2021/GDW-Metadata/metadata/Logs/Logs_02-2021/11-02/D11-Messages.xls", path "/Volumes/CentralDataCache/2021/GDW-Metadata/metadata/Logs/Logs_02-2021/12-02/D12-Messages.xls", path "/Volumes/CentralDataCache/2021/GDW-Metadata/metadata/Logs/Logs_02-2021/13-02/D13-Messages.xls", path "/Volumes/CentralDataCache/2021/GDW-Metadata/metadata/Logs/Logs_02-2021/14-02/D14-Messages.xls", path "/Volumes/CentralDataCache/2021/GDW-Metadata/metadata/Logs/Logs_02-2021/15-02/D15-Messages.xls", path "/Volumes/CentralDataCache/2021/GDW-Metadata/metadata/Logs/Logs_02-2021/16-02/D16-Messages.xls", path "/Volumes/CentralDataCache/2021/GDW-Metadata/metadata/Logs/Logs_02-2021/17-02/D17-Messages.xls", path "/Volumes/CentralDataCache/2021/GDW-Metadata/metadata/Logs/Logs_02-2021/18-02/D18-Messages.xls", path "/Volumes/CentralDataCache/2021/GDW-Metadata/metadata/Logs/Logs_02-2021/19-02/D19-Messages.xls", path "/Volumes/CentralDataCache/2021/GDW-Metadata/metadata/Logs/Logs_02-2021/20-02/D20-Messages.xls", path "/Volumes/CentralDataCache/2021/GDW-Metadata/metadata/Logs/Logs_02-2021/21-02/D21-Messages.xls", path "/Volumes/CentralDataCache/2021/GDW-Metadata/metadata/Logs/Logs_02-2021/22-02/D22-Messages.xls", path "/Volumes/CentralDataCache/2021/GDW-Metadata/metadata/Logs/Logs_02-2021/23-02/D23-Messages.xls", path "/Volumes/CentralDataCache/2021/GDW-Metadata/metadata/Logs/Logs_02-2021/24-02/D24-Messages.xls", path "/Volumes/CentralDataCache/2021/GDW-Metadata/metadata/Logs/Logs_02-2021/25-02/D25-Messages.xls", path "/Volumes/CentralDataCache/2021/GDW-Metadata/metadata/Logs/Logs_02-2021/26-02/D26-Messages.xls", path "/Volumes/CentralDataCache/2021/GDW-Metadata/metadata/Logs/Logs_02-2021/27-02/D27-Messages.xls", path "/Volumes/CentralDataCache/2021/GDW-Metadata/metadata/Logs/Logs_02-2021/28-02/D28-Messages.xls", path "/Volumes/CentralDataCache/2021/GDW-Metadata/metadata/Logs/Logs_03-2021/01-03/D01-Messages.xls", path "/Volumes/CentralDataCache/2021/GDW-Metadata/metadata/Logs/Logs_03-2021/02-03/D02-Messages.xls", path "/Volumes/CentralDataCache/2021/GDW-Metadata/metadata/Logs/Logs_03-2021/03-03/D03-Messages.xls", path "/Volumes/CentralDataCache/2021/GDW-Metadata/metadata/Logs/Logs_03-2021/04-03/D04-Messages.xls", path "/Volumes/CentralDataCache/2021/GDW-Metadata/metadata/Logs/Logs_03-2021/05-03/D05-Messages.xls", path "/Volumes/CentralDataCache/2021/GDW-Metadata/metadata/Logs/Logs_03-2021/06-03/D06-Messages.xls", path "/Volumes/CentralDataCache/2021/GDW-Metadata/metadata/Logs/Logs_03-2021/07-03/D07-Messages.xls", path "/Volumes/CentralDataCache/2021/GDW-Metadata/metadata/Logs/Logs_03-2021/08-03/D08-Messages.xls", path "/Volumes/CentralDataCache/2021/GDW-Metadata/metadata/Logs/Logs_03-2021/09-03/D09-Messages.xls", path "/Volumes/CentralDataCache/2021/GDW-Metadata/metadata/Logs/Logs_03-2021/10-03/D10-Messages.xls", path "/Volumes/CentralDataCache/2021/GDW-Metadata/metadata/Logs/Logs_03-2021/11-03/D11-Messages.xls", path "/Volumes/CentralDataCache/2021/GDW-Metadata/metadata/Logs/Logs_03-2021/12-03/D12-Messages.xls", path "/Volumes/CentralDataCache/2021/GDW-Metadata/metadata/Logs/Logs_03-2021/13-03/D13-Messages.xls", path "/Volumes/CentralDataCache/2021/GDW-Metadata/metadata/Logs/Logs_03-2021/14-03/D14-Messages.xls", path "/Volumes/CentralDataCache/2021/GDW-Metadata/metadata/Logs/Logs_03-2021/15-03/D15-Messages.xls", path "/Volumes/CentralDataCache/2021/GDW-Metadata/metadata/Logs/Logs_03-2021/16-03/D16-Messages.xls", path "/Volumes/CentralDataCache/2021/GDW-Metadata/metadata/Logs/Logs_03-2021/17-03/D17-Messages.xls", path "/Volumes/CentralDataCache/2021/GDW-Metadata/metadata/Logs/Logs_03-2021/18-03/D18-Messages.xls", path "/Volumes/CentralDataCache/2021/GDW-Metadata/metadata/Logs/Logs_03-2021/19-03/D19-Messages.xls", path "/Volumes/CentralDataCache/2021/GDW-Metadata/metadata/Logs/Logs_03-2021/20-03/D20-Messages.xls", path "/Volumes/CentralDataCache/2021/GDW-Metadata/metadata/Logs/Logs_03-2021/21-03/D21-Messages.xls", path "/Volumes/CentralDataCache/2021/GDW-Metadata/metadata/Logs/Logs_03-2021/22-03/D22-Messages.xls", path "/Volumes/CentralDataCache/2021/GDW-Metadata/metadata/Logs/Logs_03-2021/23-03/D23-Messages.xls", path "/Volumes/CentralDataCache/2021/GDW-Metadata/metadata/Logs/Logs_03-2021/24-03/D24-Messages.xls", path "/Volumes/CentralDataCache/2021/GDW-Metadata/metadata/Logs/Logs_03-2021/25-03/D25-Messages.xls", path "/Volumes/CentralDataCache/2021/GDW-Metadata/metadata/Logs/Logs_03-2021/26-03/D26-Messages.xls", path "/Volumes/CentralDataCache/2021/GDW-Metadata/metadata/Logs/Logs_03-2021/27-03/D27-Messages.xls", path "/Volumes/CentralDataCache/2021/GDW-Metadata/metadata/Logs/Logs_03-2021/29-03/D29-Messages.xls", path "/Volumes/CentralDataCache/2021/GDW-Metadata/metadata/Logs/Logs_03-2021/30-03/D30-Messages.xls", path "/Volumes/CentralDataCache/2021/GDW-Metadata/metadata/Logs/Logs_03-2021/31-03/D31-Messages.xls", path "/Volumes/CentralDataCache/2021/GDW-Metadata/metadata/Logs/Logs_04-2021/01-04/D01-Messages.xls", path "/Volumes/CentralDataCache/2021/GDW-Metadata/metadata/Logs/Logs_04-2021/02-04/D02-Messages.xls", path "/Volumes/CentralDataCache/2021/GDW-Metadata/metadata/Logs/Logs_04-2021/03-04/D03-Messages.xls", path "/Volumes/CentralDataCache/2021/GDW-Metadata/metadata/Logs/Logs_04-2021/04-04/D04-Messages.xls", path "/Volumes/CentralDataCache/2021/GDW-Metadata/metadata/Logs/Logs_04-2021/05-04/D05-Messages.xls", path "/Volumes/CentralDataCache/2021/GDW-Metadata/metadata/Logs/Logs_04-2021/06-04/D06-Messages.xls", path "/Volumes/CentralDataCache/2021/GDW-Metadata/metadata/Logs/Logs_04-2021/07-04/D07-Messages.xls", path "/Volumes/CentralDataCache/2021/GDW-Metadata/metadata/Logs/Logs_04-2021/08-04/D08-Messages.xls", path "/Volumes/CentralDataCache/2021/GDW-Metadata/metadata/Logs/Logs_04-2021/09-04/D09-Messages.xls", path "/Volumes/CentralDataCache/2021/GDW-Metadata/metadata/Logs/Logs_04-2021/10-04/D10-Messages.xls", path "/Volumes/CentralDataCache/2021/GDW-Metadata/metadata/Logs/Logs_04-2021/11-04/D11-Messages.xls", path "/Volumes/CentralDataCache/2021/GDW-Metadata/metadata/Logs/Logs_04-2021/12-04/D12-Messages.xls", path "/Volumes/CentralDataCache/2021/GDW-Metadata/metadata/Logs/Logs_04-2021/13-04/D13-Messages.xls", path "/Volumes/CentralDataCache/2021/GDW-Metadata/metadata/Logs/Logs_04-2021/14-04/D14-Messages.xls", path "/Volumes/CentralDataCache/2021/GDW-Metadata/metadata/Logs/Logs_04-2021/15-04/D15-Messages.xls", path "/Volumes/CentralDataCache/2021/GDW-Metadata/metadata/Logs/Logs_04-2021/16-04/D16-Messages.xls", path "/Volumes/CentralDataCache/2021/GDW-Metadata/metadata/Logs/Logs_04-2021/17-04/D17-Messages.xls", path "/Volumes/CentralDataCache/2021/GDW-Metadata/metadata/Logs/Logs_04-2021/18-04/D18-Messages.xls", path "/Volumes/CentralDataCache/2021/GDW-Metadata/metadata/Logs/Logs_04-2021/19-04/D19-Messages.xls", path "/Volumes/CentralDataCache/2021/GDW-Metadata/metadata/Logs/Logs_04-2021/20-04/D20-Messages.xls", path "/Volumes/CentralDataCache/2021/GDW-Metadata/metadata/Logs/Logs_04-2021/21-04/D21-Messages.xls", path "/Volumes/CentralDataCache/2021/GDW-Metadata/metadata/Logs/Logs_04-2021/22-04/D22-Messages.xls", path "/Volumes/CentralDataCache/2021/GDW-Metadata/metadata/Logs/Logs_04-2021/23-04/D23-Messages.xls", path "/Volumes/CentralDataCache/2021/GDW-Metadata/metadata/Logs/Logs_04-2021/24-04/D24-Messages.xls", path "/Volumes/CentralDataCache/2021/GDW-Metadata/metadata/Logs/Logs_04-2021/25-04/D25-Messages.xls", path "/Volumes/CentralDataCache/2021/GDW-Metadata/metadata/Logs/Logs_04-2021/26-04/D26-Messages.xls", path "/Volumes/CentralDataCache/2021/GDW-Metadata/metadata/Logs/Logs_04-2021/27-04/D27-Messages.xls", path "/Volumes/CentralDataCache/2021/GDW-Metadata/metadata/Logs/Logs_04-2021/28-04/D28-Messages.xls", path "/Volumes/CentralDataCache/2021/GDW-Metadata/metadata/Logs/Logs_04-2021/29-04/D29-Messages.xls", path "/Volumes/CentralDataCache/2021/GDW-Metadata/metadata/Logs/Logs_04-2021/30-04/D30-Messages.xls", path "/Volumes/CentralDataCache/2021/GDW-Metadata/metadata/Logs/Logs_05-2021/01-05/D01-Messages.xls", path "/Volumes/CentralDataCache/2021/GDW-Metadata/metadata/Logs/Logs_05-2021/02-05/D02-Messages.xls", path "/Volumes/CentralDataCache/2021/GDW-Metadata/metadata/Logs/Logs_05-2021/03-05/D03-Messages.xls", path "/Volumes/CentralDataCache/2021/GDW-Metadata/metadata/Logs/Logs_05-2021/04-05/D04-Messages.xls", path "/Volumes/CentralDataCache/2021/GDW-Metadata/metadata/Logs/Logs_05-2021/05-05/D05-Messages.xls", path "/Volumes/CentralDataCache/2021/GDW-Metadata/metadata/Logs/Logs_05-2021/06-05/D06-Messages.xls", path "/Volumes/CentralDataCache/2021/GDW-Metadata/metadata/Logs/Logs_05-2021/07-05/D07-Messages.xls", path "/Volumes/CentralDataCache/2021/GDW-Metadata/metadata/Logs/Logs_05-2021/08-05/D08-Messages.xls", path "/Volumes/CentralDataCache/2021/GDW-Metadata/metadata/Logs/Logs_05-2021/09-05/D09-Messages.xls", path "/Volumes/CentralDataCache/2021/GDW-Metadata/metadata/Logs/Logs_05-2021/10-05/D10-Messages.xls", path "/Volumes/CentralDataCache/2021/GDW-Metadata/metadata/Logs/Logs_05-2021/11-05/D11-Messages.xls", path "/Volumes/CentralDataCache/2021/GDW-Metadata/metadata/Logs/Logs_05-2021/12-05/D12-Messages.xls", path "/Volumes/CentralDataCache/2021/GDW-Metadata/metadata/Logs/Logs_05-2021/13-05/D13-Messages.xls", path "/Volumes/CentralDataCache/2021/GDW-Metadata/metadata/Logs/Logs_05-2021/14-05/D14-Messages.xls", path "/Volumes/CentralDataCache/2021/GDW-Metadata/metadata/Logs/Logs_05-2021/15-05/D15-Messages.xls", path "/Volumes/CentralDataCache/2021/GDW-Metadata/metadata/Logs/Logs_05-2021/16-05/D16-Messages.xls", path "/Volumes/CentralDataCache/2021/GDW-Metadata/metadata/Logs/Logs_05-2021/17-05/D17-Messages.xls", path "/Volumes/CentralDataCache/2021/GDW-Metadata/metadata/Logs/Logs_05-2021/18-05/D18-Messages.xls", path "/Volumes/CentralDataCache/2021/GDW-Metadata/metadata/Logs/Logs_05-2021/19-05/D19-Messages.xls", path "/Volumes/CentralDataCache/2021/GDW-Metadata/metadata/Logs/Logs_05-2021/20-05/D20-Messages.xls", path "/Volumes/CentralDataCache/2021/GDW-Metadata/metadata/Logs/Logs_05-2021/21-05/D21-Messages.xls", path "/Volumes/CentralDataCache/2021/GDW-Metadata/metadata/Logs/Logs_05-2021/22-05/D22-Messages.xls", path "/Volumes/CentralDataCache/2021/GDW-Metadata/metadata/Logs/Logs_05-2021/23-05/D23-Messages.xls", path "/Volumes/CentralDataCache/2021/GDW-Metadata/metadata/Logs/Logs_05-2021/24-05/D24-Messages.xls", path "/Volumes/CentralDataCache/2021/GDW-Metadata/metadata/Logs/Logs_05-2021/25-05/D25-Messages.xls", path "/Volumes/CentralDataCache/2021/GDW-Metadata/metadata/Logs/Logs_05-2021/26-05/D26-Messages.xls", path "/Volumes/CentralDataCache/2021/GDW-Metadata/metadata/Logs/Logs_05-2021/27-05/D27-Messages.xls", path "/Volumes/CentralDataCache/2021/GDW-Metadata/metadata/Logs/Logs_05-2021/28-05/D28-Messages.xls", path "/Volumes/CentralDataCache/2021/GDW-Metadata/metadata/Logs/Logs_05-2021/29-05/D29-Messages.xls", path "/Volumes/CentralDataCache/2021/GDW-Metadata/metadata/Logs/Logs_05-2021/30-05/D30-Messages.xls", path "/Volumes/CentralDataCache/2021/GDW-Metadata/metadata/Logs/Logs_05-2021/31-05/D31-Messages.xls", path "/Volumes/CentralDataCache/2021/GDW-Metadata/metadata/Logs/Logs_06-2021/01-06/D01-Messages.xls", path "/Volumes/CentralDataCache/2021/GDW-Metadata/metadata/Logs/Logs_06-2021/02-06/D02-Messages.xls", path "/Volumes/CentralDataCache/2021/GDW-Metadata/metadata/Logs/Logs_06-2021/03-06/D03-Messages.xls", path "/Volumes/CentralDataCache/2021/GDW-Metadata/metadata/Logs/Logs_06-2021/04-06/D04-Messages.xls", path "/Volumes/CentralDataCache/2021/GDW-Metadata/metadata/Logs/Logs_06-2021/05-06/D05-Messages.xls", path "/Volumes/CentralDataCache/2021/GDW-Metadata/metadata/Logs/Logs_06-2021/06-06/D06-Messages.xls", path "/Volumes/CentralDataCache/2021/GDW-Metadata/metadata/Logs/Logs_06-2021/07-06/D07-Messages.xls", path "/Volumes/CentralDataCache/2021/GDW-Metadata/metadata/Logs/Logs_06-2021/08-06/D08-Messages.xls", path "/Volumes/CentralDataCache/2021/GDW-Metadata/metadata/Logs/Logs_06-2021/09-06/D09-Messages.xls", path "/Volumes/CentralDataCache/2021/GDW-Metadata/metadata/Logs/Logs_06-2021/10-06/D10-Messages.xls", path "/Volumes/CentralDataCache/2021/GDW-Metadata/metadata/Logs/Logs_06-2021/11-06/D11-Messages.xls", path "/Volumes/CentralDataCache/2021/GDW-Metadata/metadata/Logs/Logs_06-2021/12-06/D12-Messages.xls", path "/Volumes/CentralDataCache/2021/GDW-Metadata/metadata/Logs/Logs_06-2021/13-06/D13-Messages.xls", path "/Volumes/CentralDataCache/2021/GDW-Metadata/metadata/Logs/Logs_06-2021/14-06/D14-Messages.xls", path "/Volumes/CentralDataCache/2021/GDW-Metadata/metadata/Logs/Logs_06-2021/15-06/D15-Messages.xls", path "/Volumes/CentralDataCache/2021/GDW-Metadata/metadata/Logs/Logs_06-2021/16-06/D16-Messages.xls", path "/Volumes/CentralDataCache/2021/GDW-Metadata/metadata/Logs/Logs_06-2021/17-06/D17-Messages.xls", path "/Volumes/CentralDataCache/2021/GDW-Metadata/metadata/Logs/Logs_06-2021/18-06/D18-Messages.xls", path "/Volumes/CentralDataCache/2021/GDW-Metadata/metadata/Logs/Logs_06-2021/19-06/D19-Messages.xls", path "/Volumes/CentralDataCache/2021/GDW-Metadata/metadata/Logs/Logs_06-2021/20-06/D20-Messages.xls", path "/Volumes/CentralDataCache/2021/GDW-Metadata/metadata/Logs/Logs_06-2021/21-06/D21-Messages.xls", path "/Volumes/CentralDataCache/2021/GDW-Metadata/metadata/Logs/Logs_06-2021/22-06/D22-Messages.xls", path "/Volumes/CentralDataCache/2021/GDW-Metadata/metadata/Logs/Logs_06-2021/23-06/D23-Messages.xls", path "/Volumes/CentralDataCache/2021/GDW-Metadata/metadata/Logs/Logs_06-2021/24-06/D24-Messages.xls", path "/Volumes/CentralDataCache/2021/GDW-Metadata/metadata/Logs/Logs_06-2021/25-06/D25-Messages.xls", path "/Volumes/CentralDataCache/2021/GDW-Metadata/metadata/Logs/Logs_06-2021/26-06/D26-Messages.xls", path "/Volumes/CentralDataCache/2021/GDW-Metadata/metadata/Logs/Logs_06-2021/27-06/D27-Messages.xls", path "/Volumes/CentralDataCache/2021/GDW-Metadata/metadata/Logs/Logs_06-2021/28-06/D28-Messages.xls", path "/Volumes/CentralDataCache/2021/GDW-Metadata/metadata/Logs/Logs_06-2021/29-06/D29-Messages.xls", path "/Volumes/CentralDataCache/2021/GDW-Metadata/metadata/Logs/Logs_06-2021/30-06/D30-Messages.xls", path "/Volumes/CentralDataCache/2021/GDW-Metadata/metadata/Logs/Logs_07-2021/01-07/D01-Messages.xls", path "/Volumes/CentralDataCache/2021/GDW-Metadata/metadata/Logs/Logs_07-2021/02-07/D02-Messages.xls", path "/Volumes/CentralDataCache/2021/GDW-Metadata/metadata/Logs/Logs_07-2021/03-07/D03-Messages.xls", path "/Volumes/CentralDataCache/2021/GDW-Metadata/metadata/Logs/Logs_07-2021/04-07/D04-Messages.xls", path "/Volumes/CentralDataCache/2021/GDW-Metadata/metadata/Logs/Logs_07-2021/05-07/D05-Messages.xls", path "/Volumes/CentralDataCache/2021/GDW-Metadata/metadata/Logs/Logs_07-2021/06-07/D06-Messages.xls", path "/Volumes/CentralDataCache/2021/GDW-Metadata/metadata/Logs/Logs_07-2021/07-07/D07-Messages.xls", path "/Volumes/CentralDataCache/2021/GDW-Metadata/metadata/Logs/Logs_07-2021/08-07/D08-Messages.xls", path "/Volumes/CentralDataCache/2021/GDW-Metadata/metadata/Logs/Logs_07-2021/09-07/D09-Messages.xls", path "/Volumes/CentralDataCache/2021/GDW-Metadata/metadata/Logs/Logs_07-2021/10-07/D10-Messages.xls", path "/Volumes/CentralDataCache/2021/GDW-Metadata/metadata/Logs/Logs_07-2021/11-07/D11-Messages.xls", path "/Volumes/CentralDataCache/2021/GDW-Metadata/metadata/Logs/Logs_07-2021/12-07/D12-Messages.xls", path "/Volumes/CentralDataCache/2021/GDW-Metadata/metadata/Logs/Logs_07-2021/13-07/D13-Messages.xls", path "/Volumes/CentralDataCache/2021/GDW-Metadata/metadata/Logs/Logs_07-2021/14-07/D14-Messages.xls", path "/Volumes/CentralDataCache/2021/GDW-Metadata/metadata/Logs/Logs_07-2021/15-07/D15-Messages.xls", path "/Volumes/CentralDataCache/2021/GDW-Metadata/metadata/Logs/Logs_07-2021/16-07/D16-Messages.xls", path "/Volumes/CentralDataCache/2021/GDW-Metadata/metadata/Logs/Logs_07-2021/17-07/D17-Messages.xls", path "/Volumes/CentralDataCache/2021/GDW-Metadata/metadata/Logs/Logs_07-2021/18-07/D18-Messages.xls", path "/Volumes/CentralDataCache/2021/GDW-Metadata/metadata/Logs/Logs_07-2021/19-07/D19-Messages.xls", path "/Volumes/CentralDataCache/2021/GDW-Metadata/metadata/Logs/Logs_07-2021/20-07/D20-Messages.xls", path "/Volumes/CentralDataCache/2021/GDW-Metadata/metadata/Logs/Logs_07-2021/21-07/D21-Messages.xls", path "/Volumes/CentralDataCache/2021/GDW-Metadata/metadata/Logs/Logs_07-2021/22-07/D22-Messages.xls", path "/Volumes/CentralDataCache/2021/GDW-Metadata/metadata/Logs/Logs_07-2021/23-07/D23-Messages.xls", path "/Volumes/CentralDataCache/2021/GDW-Metadata/metadata/Logs/Logs_07-2021/24-07/D24-Messages.xls", path "/Volumes/CentralDataCache/2021/GDW-Metadata/metadata/Logs/Logs_07-2021/25-07/D25-Messages.xls", path "/Volumes/CentralDataCache/2021/GDW-Metadata/metadata/Logs/Logs_07-2021/26-07/D26-Messages.xls", path "/Volumes/CentralDataCache/2021/GDW-Metadata/metadata/Logs/Logs_07-2021/27-07/D27-Messages.xls", path "/Volumes/CentralDataCache/2021/GDW-Metadata/metadata/Logs/Logs_07-2021/28-07/D28-Messages.xls", path "/Volumes/CentralDataCache/2021/GDW-Metadata/metadata/Logs/Logs_07-2021/29-07/D29-Messages.xls", path "/Volumes/CentralDataCache/2021/GDW-Metadata/metadata/Logs/Logs_07-2021/30-07/D30-Messages.xls", path "/Volumes/CentralDataCache/2021/GDW-Metadata/metadata/Logs/Logs_07-2021/31-07/D31-Messages.xls", path "/Volumes/CentralDataCache/2021/GDW-Metadata/metadata/Logs/Logs_08-2021/01-08/D01-Messages.xls", path "/Volumes/CentralDataCache/2021/GDW-Metadata/metadata/Logs/Logs_08-2021/02-08/D02-Messages.xls", path "/Volumes/CentralDataCache/2021/GDW-Metadata/metadata/Logs/Logs_08-2021/03-08/D03-Messages.xls", path "/Volumes/CentralDataCache/2021/GDW-Metadata/metadata/Logs/Logs_08-2021/04-08/D04-Messages.xls", path "/Volumes/CentralDataCache/2021/GDW-Metadata/metadata/Logs/Logs_08-2021/05-08/D05-Messages.xls", path "/Volumes/CentralDataCache/2021/GDW-Metadata/metadata/Logs/Logs_08-2021/06-08/D06-Messages.xls", path "/Volumes/CentralDataCache/2021/GDW-Metadata/metadata/Logs/Logs_08-2021/07-08/D07-Messages.xls", path "/Volumes/CentralDataCache/2021/GDW-Metadata/metadata/Logs/Logs_08-2021/08-08/D08-Messages.xls", path "/Volumes/CentralDataCache/2021/GDW-Metadata/metadata/Logs/Logs_08-2021/09-08/D09-Messages.xls", path "/Volumes/CentralDataCache/2021/GDW-Metadata/metadata/Logs/Logs_08-2021/10-08/D10-Messages.xls", path "/Volumes/CentralDataCache/2021/GDW-Metadata/metadata/Logs/Logs_08-2021/11-08/D11-Messages.xls", path "/Volumes/CentralDataCache/2021/GDW-Metadata/metadata/Logs/Logs_08-2021/12-08/D12-Messages.xls", path "/Volumes/CentralDataCache/2021/GDW-Metadata/metadata/Logs/Logs_08-2021/13-08/D13-Messages.xls", path "/Volumes/CentralDataCache/2021/GDW-Metadata/metadata/Logs/Logs_08-2021/17-08/D17-Messages.xls", path "/Volumes/CentralDataCache/2021/GDW-Metadata/metadata/Logs/Logs_08-2021/18-08/D18-Messages.xls", path "/Volumes/CentralDataCache/2021/GDW-Metadata/metadata/Logs/Logs_08-2021/19-08/D19-Messages.xls", path "/Volumes/CentralDataCache/2021/GDW-Metadata/metadata/Logs/Logs_08-2021/20-08/D20-Messages.xls", path "/Volumes/CentralDataCache/2021/GDW-Metadata/metadata/Logs/Logs_08-2021/21-08/D21-Messages.xls", path "/Volumes/CentralDataCache/2021/GDW-Metadata/metadata/Logs/Logs_08-2021/22-08/D22-Messages.xls", path "/Volumes/CentralDataCache/2021/GDW-Metadata/metadata/Logs/Logs_08-2021/23-08/D23-Messages.xls", path "/Volumes/CentralDataCache/2021/GDW-Metadata/metadata/Logs/Logs_08-2021/24-08/D24-Messages.xls", path "/Volumes/CentralDataCache/2021/GDW-Metadata/metadata/Logs/Logs_08-2021/25-08/D25-Messages.xls", path "/Volumes/CentralDataCache/2021/GDW-Metadata/metadata/Logs/Logs_08-2021/26-08/D26-Messages.xls", path "/Volumes/CentralDataCache/2021/GDW-Metadata/metadata/Logs/Logs_08-2021/27-08/D27-Messages.xls", path "/Volumes/CentralDataCache/2021/GDW-Metadata/metadata/Logs/Logs_08-2021/28-08/D28-Messages.xls", path "/Volumes/CentralDataCache/2021/GDW-Metadata/metadata/Logs/Logs_08-2021/29-08/D29-Messages.xls", path "/Volumes/CentralDataCache/2021/GDW-Metadata/metadata/Logs/Logs_08-2021/30-08/D30-Messages.xls", path "/Volumes/CentralDataCache/2021/GDW-Metadata/metadata/Logs/Logs_08-2021/31-08/D31-Messages.xls", path "/Volumes/CentralDataCache/2021/GDW-Metadata/metadata/Logs/Logs_09-2021/01-09/D01-Messages.xls", path "/Volumes/CentralDataCache/2021/GDW-Metadata/metadata/Logs/Logs_09-2021/02-09/D02-Messages.xls", path "/Volumes/CentralDataCache/2021/GDW-Metadata/metadata/Logs/Logs_09-2021/03-09/D03-Messages.xls", path "/Volumes/CentralDataCache/2021/GDW-Metadata/metadata/Logs/Logs_09-2021/04-09/D04-Messages.xls", path "/Volumes/CentralDataCache/2021/GDW-Metadata/metadata/Logs/Logs_09-2021/05-09/D05-Messages.xls", path "/Volumes/CentralDataCache/2021/GDW-Metadata/metadata/Logs/Logs_09-2021/06-09/D06-Messages.xls", path "/Volumes/CentralDataCache/2021/GDW-Metadata/metadata/Logs/Logs_09-2021/07-09/D07-Messages.xls", path "/Volumes/CentralDataCache/2021/GDW-Metadata/metadata/Logs/Logs_09-2021/08-09/D08-Messages.xls", path "/Volumes/CentralDataCache/2021/GDW-Metadata/metadata/Logs/Logs_09-2021/09-09/D09-Messages.xls", path "/Volumes/CentralDataCache/2021/GDW-Metadata/metadata/Logs/Logs_09-2021/10-09/D10-Messages.xls", path "/Volumes/CentralDataCache/2021/GDW-Metadata/metadata/Logs/Logs_09-2021/11-09/D11-Messages.xls", path "/Volumes/CentralDataCache/2021/GDW-Metadata/metadata/Logs/Logs_09-2021/12-09/D12-Messages.xls", path "/Volumes/CentralDataCache/2021/GDW-Metadata/metadata/Logs/Logs_09-2021/13-09/D13-Messages.xls", path "/Volumes/CentralDataCache/2021/GDW-Metadata/metadata/Logs/Logs_09-2021/14-09/D14-Messages.xls", path "/Volumes/CentralDataCache/2021/GDW-Metadata/metadata/Logs/Logs_09-2021/15-09/D15-Messages.xls", path "/Volumes/CentralDataCache/2021/GDW-Metadata/metadata/Logs/Logs_09-2021/16-09/D16-Messages.xls", path "/Volumes/CentralDataCache/2021/GDW-Metadata/metadata/Logs/Logs_09-2021/17-09/D17-Messages.xls", path "/Volumes/CentralDataCache/2021/GDW-Metadata/metadata/Logs/Logs_09-2021/18-09/D18-Messages.xls", path "/Volumes/CentralDataCache/2021/GDW-Metadata/metadata/Logs/Logs_09-2021/19-09/D19-Messages.xls", path "/Volumes/CentralDataCache/2021/GDW-Metadata/metadata/Logs/Logs_09-2021/20-09/D20-Messages.xls", path "/Volumes/CentralDataCache/2021/GDW-Metadata/metadata/Logs/Logs_09-2021/21-09/D21-Messages.xls", path "/Volumes/CentralDataCache/2021/GDW-Metadata/metadata/Logs/Logs_09-2021/22-09/D22-Messages.xls", path "/Volumes/CentralDataCache/2021/GDW-Metadata/metadata/Logs/Logs_09-2021/23-09/D23-Messages.xls", path "/Volumes/CentralDataCache/2021/GDW-Metadata/metadata/Logs/Logs_09-2021/24-09/D24-Messages.xls", path "/Volumes/CentralDataCache/2021/GDW-Metadata/metadata/Logs/Logs_09-2021/25-09/D25-Messages.xls", path "/Volumes/CentralDataCache/2021/GDW-Metadata/metadata/Logs/Logs_09-2021/26-09/D26-Messages.xls", path "/Volumes/CentralDataCache/2021/GDW-Metadata/metadata/Logs/Logs_09-2021/27-09/D27-Messages.xls", path "/Volumes/CentralDataCache/2021/GDW-Metadata/metadata/Logs/Logs_09-2021/28-09/D28-Messages.xls", path "/Volumes/CentralDataCache/2021/GDW-Metadata/metadata/Logs/Logs_09-2021/29-09/D29-Messages.xls", path "/Volumes/CentralDataCache/2021/GDW-Metadata/metadata/Logs/Logs_09-2021/30-09/D30-Messages.xls", path "/Volumes/CentralDataCache/2021/GDW-Metadata/metadata/Logs/Logs_10-2021/01-10/D01-Messages.xls", path "/Volumes/CentralDataCache/2021/GDW-Metadata/metadata/Logs/Logs_10-2021/02-10/D02-Messages.xls", path "/Volumes/CentralDataCache/2021/GDW-Metadata/metadata/Logs/Logs_10-2021/03-10/D03-Messages.xls", path "/Volumes/CentralDataCache/2021/GDW-Metadata/metadata/Logs/Logs_10-2021/04-10/D04-Messages.xls", path "/Volumes/CentralDataCache/2021/GDW-Metadata/metadata/Logs/Logs_10-2021/05-10/D05-Messages.xls", path "/Volumes/CentralDataCache/2021/GDW-Metadata/metadata/Logs/Logs_10-2021/06-10/D06-Messages.xls", path "/Volumes/CentralDataCache/2021/GDW-Metadata/metadata/Logs/Logs_10-2021/07-10/D07-Messages.xls", path "/Volumes/CentralDataCache/2021/GDW-Metadata/metadata/Logs/Logs_10-2021/08-10/D08-Messages.xls", path "/Volumes/CentralDataCache/2021/GDW-Metadata/metadata/Logs/Logs_10-2021/09-10/D09-Messages.xls", path "/Volumes/CentralDataCache/2021/GDW-Metadata/metadata/Logs/Logs_10-2021/10-10/D10-Messages.xls", path "/Volumes/CentralDataCache/2021/GDW-Metadata/metadata/Logs/Logs_10-2021/11-10/D11-Messages.xls", path "/Volumes/CentralDataCache/2021/GDW-Metadata/metadata/Logs/Logs_10-2021/12-10/D12-Messages.xls", path "/Volumes/CentralDataCache/2021/GDW-Metadata/metadata/Logs/Logs_10-2021/13-10/D13-Messages.xls", path "/Volumes/CentralDataCache/2021/GDW-Metadata/metadata/Logs/Logs_10-2021/14-10/D14-Messages.xls", path "/Volumes/CentralDataCache/2021/GDW-Metadata/metadata/Logs/Logs_10-2021/15-10/D15-Messages.xls", path "/Volumes/CentralDataCache/2021/GDW-Metadata/metadata/Logs/Logs_10-2021/16-10/D16-Messages.xls", path "/Volumes/CentralDataCache/2021/GDW-Metadata/metadata/Logs/Logs_10-2021/17-10/D17-Messages.xls", path "/Volumes/CentralDataCache/2021/GDW-Metadata/metadata/Logs/Logs_10-2021/18-10/D18-Messages.xls", path "/Volumes/CentralDataCache/2021/GDW-Metadata/metadata/Logs/Logs_10-2021/19-10/D19-Messages.xls", path "/Volumes/CentralDataCache/2021/GDW-Metadata/metadata/Logs/Logs_10-2021/20-10/D20-Messages.xls", path "/Volumes/CentralDataCache/2021/GDW-Metadata/metadata/Logs/Logs_10-2021/21-10/D21-Messages.xls", path "/Volumes/CentralDataCache/2021/GDW-Metadata/metadata/Logs/Logs_10-2021/22-10/D22-Messages.xls", path "/Volumes/CentralDataCache/2021/GDW-Metadata/metadata/Logs/Logs_10-2021/23-10/D23-Messages.xls", path "/Volumes/CentralDataCache/2021/GDW-Metadata/metadata/Logs/Logs_10-2021/24-10/D24-Messages.xls", path "/Volumes/CentralDataCache/2021/GDW-Metadata/metadata/Logs/Logs_10-2021/25-10/D25-Messages.xls", path "/Volumes/CentralDataCache/2021/GDW-Metadata/metadata/Logs/Logs_10-2021/26-10/D26-Messages.xls"] ("All Files in Dir")] -> w2
    frame False {
      n2 = call <vilib>:"Recursive File List.vi"("pattern"="*Messages.xls", "Continue Recursing on Error? (F)"=TRUE, "Folder Path"="folder Path") -> ("Number of Files"=→"Number of Files":i32, "All Files in Dir"=w4:path[])  [unwired: 4 in, 3 out]
    }
    frame True {
    }
  }
  "All Files in Dir" <- w2
